vi "JSONRPC-GetValue.vi"(10 "key":string, 11 "input string":string) -> (3 "value":string)   [LabVIEW 2013]
doc: "Searches for <b>key</b> in <b>input string</b> and returns its value (or empty string, if not found)."
uses:
  <vilib>/regexp/Match Regular Expression.xnode
panel:
  # "GetValue"
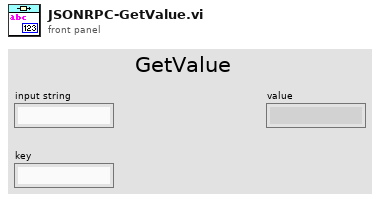
[diagram p1: front panel]
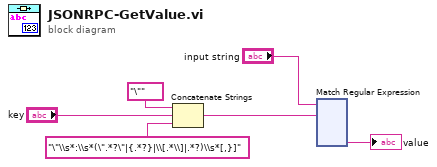
[diagram p0: block diagram]
diagram:
  n1 = Concatenate Strings("\"" ("f"), "key", "\"\\s*:\\s*(\".*?\"|{.*?}|\\[.*\\]|.*?)\\s*[,}]" ("f")) -> (w2:string)
  n2 = xnode "Match Regular Expression"("input string"="input string", "regular expression"=w2) -> ("submatch 1"=→"value":string)  [unwired: 4 in, 5 out]
